vi "Clusterwitharraypictring.vi"(1 "Cluster In":cluster{"Array In":u16[], "Ring":u16}) -> (0 "Cluster Out":cluster{"Array Out":u16[], "Ring":u16})   [LabVIEW 2011]
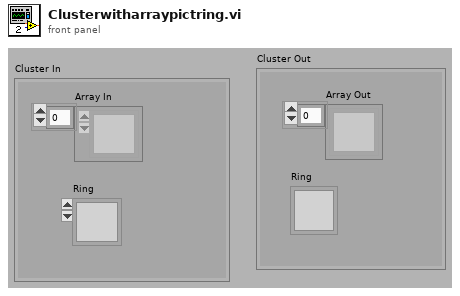
[diagram p1: front panel]
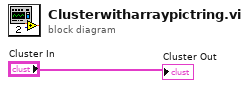
[diagram p0: block diagram]
diagram:
  "Cluster Out" <- "Cluster In"
